vi "FGV System.vi"(0 "Optionen":T2, 1 "Wartungsintervall:":sgl format="%#_5g", 2 "Zeitstempel":timestamp, 3 "Reset BMP":bool, 4 "Reset SQP":bool, 5 "error in (no error)":errorcluster caption="Fehler (Eingang, kein Fehler)", 7 "Werkseinstellung erstellen":T1 caption="Werkseinstellung", 9 "Aktionen":T3) -> (13 "Werkseinstellung erstellen":T1 caption="Werkseinstellung", 14 "Optionen":T2, 15 "Wartungsintervall:":sgl, 16 "Zeitstempel":timestamp, 17 "Reset BMP":bool, 18 "Reset SQP":bool, 19 "error out":errorcluster caption="Fehler (Ausgang)")   [LabVIEW 2020, in "System Einstellungen V2.lvlib"]
uses:
  System Einstellungen V2.lvlib
  Aktioen FGV System.ctl
  Optionen.ctl
  Visualisierungs Elemente/Button.ctl
  SysLog/SysLog Interface.ctl
  Allgemein/allgemeine Sub-VIs.lvlib
  SysLog/SysLog.lvlib
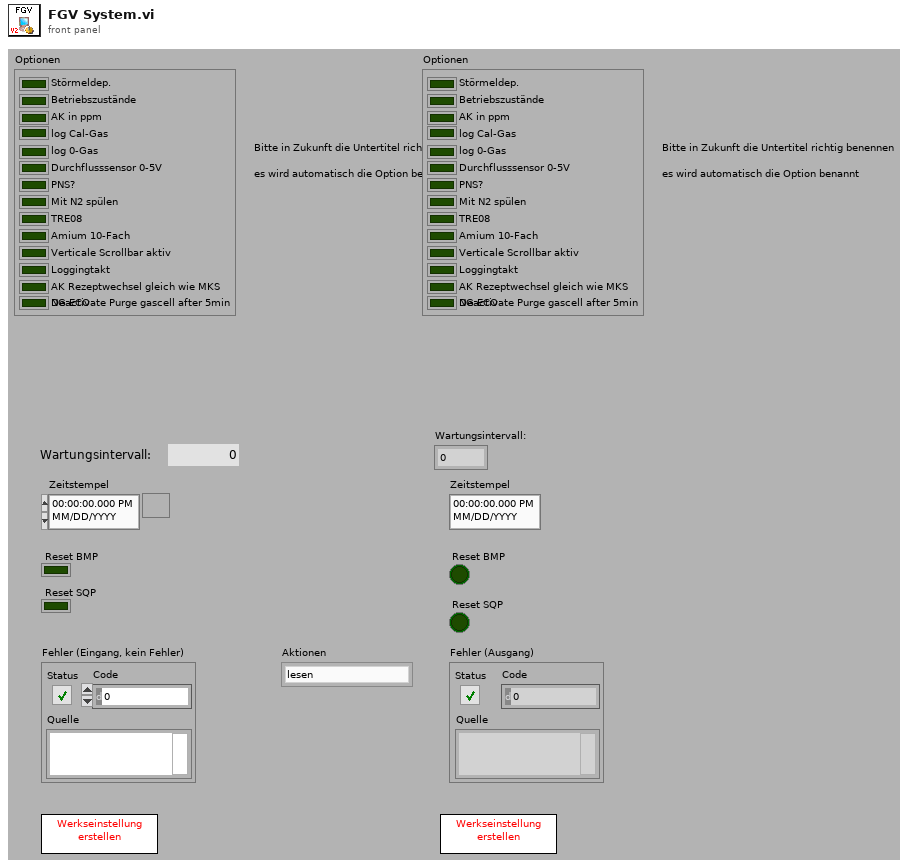
[diagram p1: front panel]
types:
  T1 = typedef "Button.ctl" = bool
  T2 = typedef "System Einstellungen V2.lvlib/Optionen.ctl" = cluster{"Störmeldep.":bool, "Betriebszustände":bool, "AK in ppm":bool, "log Cal-Gas":bool, "log 0-Gas":bool, "Durchflusssensor 0-5V":bool, "PNS?":bool, "Mit N2 spülen":bool, "TRE08":bool, "Amium 10-Fach":bool, "Verticale Scrollbar aktiv":bool, "Loggingtakt":bool, "AK Rezeptwechsel gleich wie MKS":bool, "NG ECO":bool}
  T3 = typedef "System Einstellungen V2.lvlib/Aktioen FGV System.ctl" = enum16{"lesen", "laden", "speichern", "Optionen schreiben", "Zeitstempel", "Reset BMP", "Reset SQP", "Wartung", "Werkseinstellung"}
  T4 = typedef "SysLog.lvlib/SysLog Interface.ctl" = cluster{"FehlermeldungsCode":i32, "ErfolgsmeldungsCode":i32, "ParameterListenString":string, "Anzeige":bool, "SysLogIcon":enum16{"OK", "Warnung", "Fehler"}, "intern":bool}
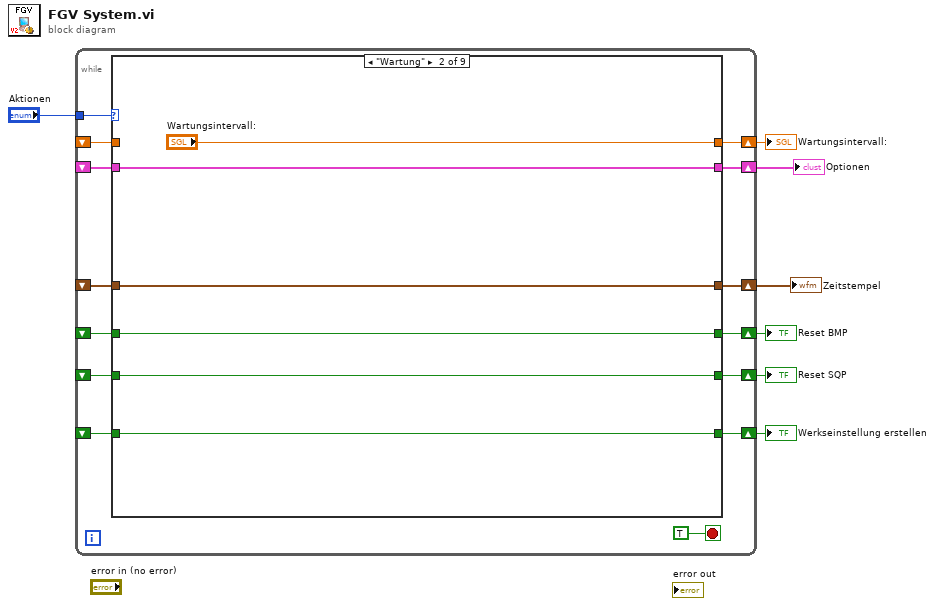
[diagram p0: block diagram]
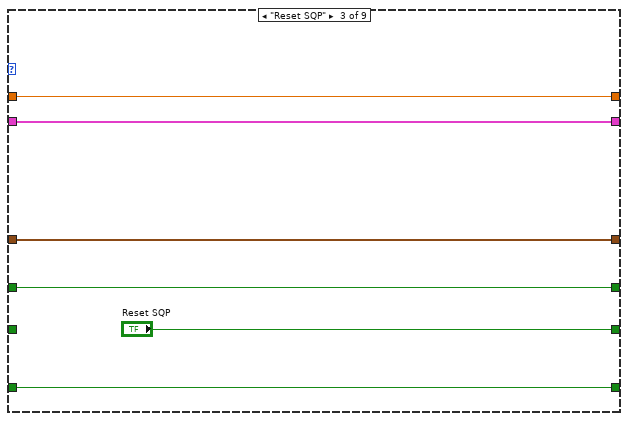
[diagram p3: hidden frame]
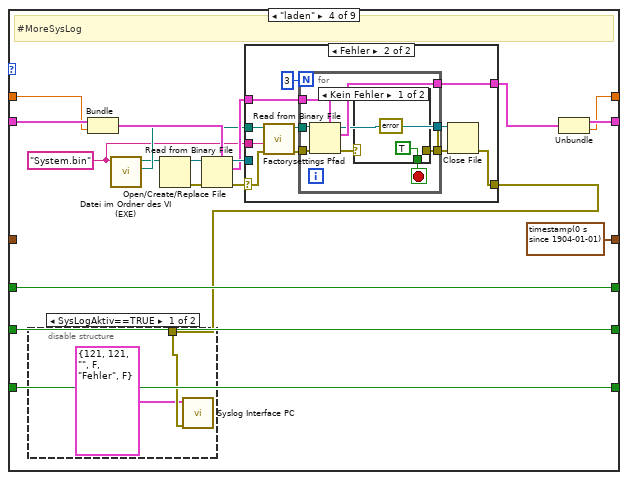
[diagram p4: hidden frame]
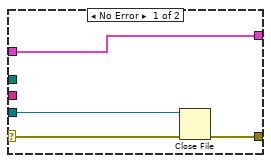
[diagram p5: hidden frame]
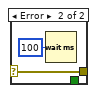
[diagram p6: hidden frame]
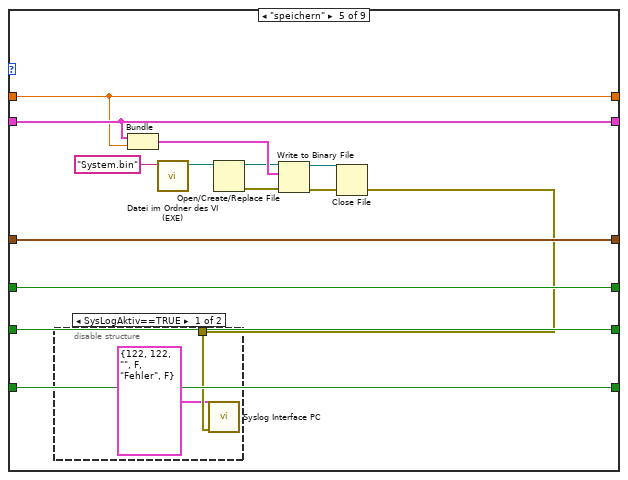
[diagram p8: hidden frame]
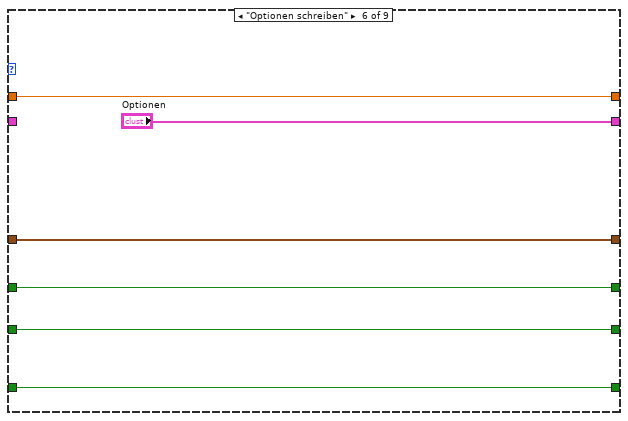
[diagram p10: hidden frame]
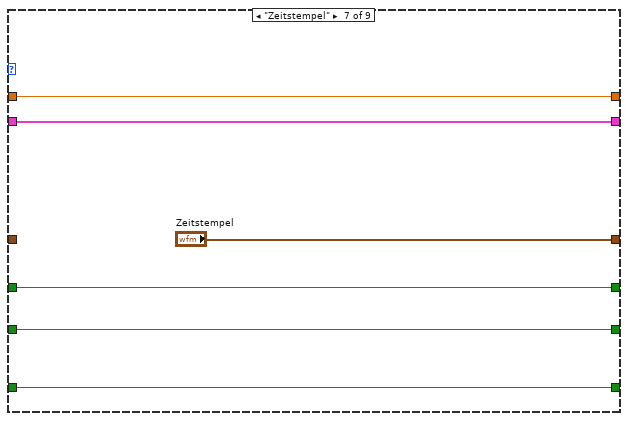
[diagram p11: hidden frame]
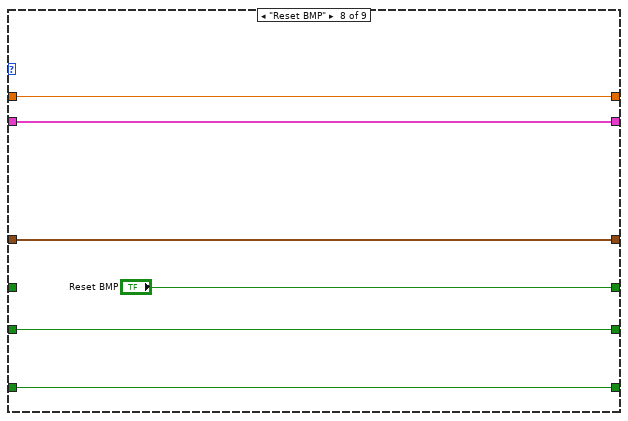
[diagram p12: hidden frame]
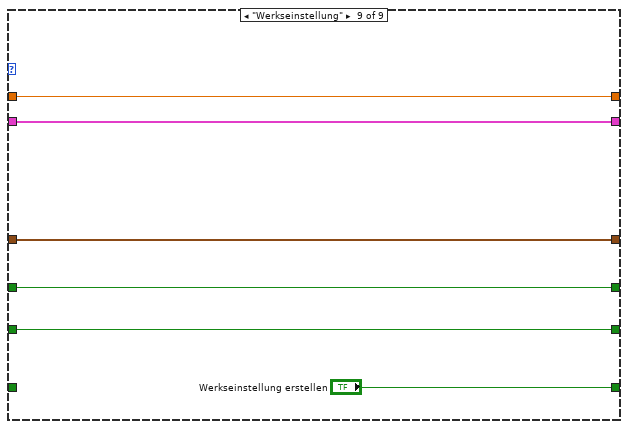
[diagram p13: hidden frame]
diagram:
  n1 = while {
    shift-right: [w18] -> w6
    shift-left: _ -> [w19]
    tunnel: "Aktionen" -> [w20]
    shift-right: [w17] -> w5
    shift-left: _ -> [w16]
    shift-right: [w15] -> w4
    shift-left: _ -> [w14]
    shift-right: [w13] -> w3
    shift-left: _ -> [w12]
    shift-right: [w11] -> w2
    shift-left: _ -> [w10]
    shift-right: [w9] -> w1
    shift-left: _ -> [w8]
    stop <- TRUE stop-if-true
    n2 = case shown="\"Wartung\"" w20 {
      tunnel: w19 -> [w27 w33 w39 w55 w96 _ w114 w121 w126]
      tunnel: [w27 w33 w39 w52 w96 "Optionen" w114 w121 w126] -> w18
      tunnel: [w26 w32 w38 timestamp(0 s since 1904-01-01) ("Zeitstempel") w100 w108 "Zeitstempel" w120 w125] -> w17
      tunnel: w16 -> [w26 w32 w38 _ w100 w108 _ w120 w125]
      tunnel: [w25 w31 w37 w57 w99 w107 w113 "Reset BMP" w124] -> w15
      tunnel: w14 -> [w25 w31 w37 w57 w99 w107 w113 _ w124]
      tunnel: [w24 w30 "Reset SQP" w56 w98 w106 w112 w118 w123] -> w13
      tunnel: w12 -> [w24 w30 _ w56 w98 w106 w112 w118 w123]
      tunnel: [w23 "Wartungsintervall:" w35 w51 w95 w105 w111 w117 w127] -> w11
      tunnel: w10 -> [w23 _ w35 w53 w95 w105 w111 w117 w127]
      tunnel: [w22 w28 w34 w40 w88 w104 w110 w116 "Werkseinstellung erstellen"] -> w9
      tunnel: w8 -> [w22 w28 w34 w40 w88 w104 w110 w116 _]
      frame "lesen", Default {
      }
      frame "Wartung" {
      }
      frame "Reset SQP" {
      }
      frame "laden" {
        w44 = "System.bin" ("Dateiname")
        # "#MoreSysLog"
        n3 = Bundle("Optionen"=w55, "Wartungsintervall:"=w53) -> (w54:cluster{"Optionen":T2, "Wartungsintervall:":sgl})  [unwired: 1 in]
        n4 = call "Datei im Ordner des VI (EXE).vi"("Dateiname"=w44) -> ("Ordner des Haupt-VIs"=w45:path, "Dateipfad im Ordner des Haupt-VIs"=w42:path)  [unwired: 8 in, 1 out]
        n5 = Open/Create/Replace File(file path (use dialog)=w42) -> (refnum out=w41:refnum<file>, error out=w43:errorcluster)  [unwired: 5 in, 1 out]
        n6 = Read from Binary File(5:w54, 8:w43, 11:w41) -> (0:w49:errorcluster, 2:w47:cluster{"Optionen":T2, "Wartungsintervall:":sgl}, 3:w48:refnum<file>)  [unwired: 4 out]
        n7 = case shown="Fehler" w49 {
          selector: w49 -> [w61 w65]
          tunnel: w45 -> [_ w66]
          tunnel: w47 -> [w62 w64]
          tunnel: [w62 w72] -> w46
          tunnel: [w59 w70] -> w50
          tunnel: w48 -> [w60 _]
          tunnel: w44 -> [_ w63]
          frame No Error {
            n8 = Close File(refnum=w60, error in=w61) -> (error out=w59:errorcluster)  [unwired: 1 out]
          }
          frame Error {
            n9 = call "Factorysettings Pfad.vi"("error in (no error)"=w65, "Dateiname"=w63, "Ordner des Haupt-VIs"=w66) -> ("error out"=w67:errorcluster, "Pfad Factorysettings"=w68:path)  [unwired: 7 in]
            n10 = for {
              N: 3 -> [_]
              tunnel: w67 -> [w79]
              tunnel: w68 -> [w78]
              tunnel: [w77] -> w72
              tunnel: [w76] -> w71
              tunnel: [w75] -> w69
              tunnel: w64 -> [w74]
              stop <- w80 stop-if-true
              n11 = Read from Binary File(5:w74, 8:w79, 11:w78) -> (0:w81:errorcluster, 2:w77:cluster{"Optionen":T2, "Wartungsintervall:":sgl}, 3:w75:refnum<file>)  [unwired: 3 in, 1 out]
              n12 = case shown="Kein Fehler" w81 {
                selector: w81 -> [_ w84]
                tunnel: [TRUE _] -> w80
                tunnel: [errorcluster {"status"=FALSE, "code"=0, "source"=""} ("error IO") w84] -> w76
                frame No Error {
                }
                frame Error {
                  n13 = Wait (ms)(milliseconds to wait=u32 100 ("Zu wartende ms")) -> ()  [unwired: 1 out]
                }
              }
            }
            n14 = Close File(refnum=w69, error in=w71) -> (error out=w70:errorcluster)  [unwired: 1 out]
          }
        }
        n15 = disable-structure shown="SysLogAktiv==TRUE" {
          disable-tunnel: w50 -> [w87 _]
          frame condition #0 (active) {
            n16 = call "Syslog Interface PC.vi"("Fehler (in)"=w87, "Cluster (in)"=T4 {"FehlermeldungsCode"=121, "ErfolgsmeldungsCode"=121, "ParameterListenString"="", "Anzeige"=FALSE, "SysLogIcon"=enum."Fehler", "intern"=FALSE}) -> ()  [unwired: 9 in, 1 out]
          }
          frame condition #1 {
          }
        }
        n17 = Unbundle(w46) -> ("Optionen"=w52:T2, "Wartungsintervall:"=w51:sgl)
      }
      frame "speichern" {
        n18 = Bundle("Optionen"=w96, "Wartungsintervall:"=w95) -> (w97:cluster{"Optionen":T2, "Wartungsintervall:":sgl})  [unwired: 1 in]
        n19 = call "Datei im Ordner des VI (EXE).vi"("Dateiname"="System.bin") -> ("Dateipfad im Ordner des Haupt-VIs"=w94:path)  [unwired: 8 in, 2 out]
        n20 = Open/Create/Replace File(file path (use dialog)=w94) -> (refnum out=w93:refnum<file>, error out=w92:errorcluster)  [unwired: 5 in, 1 out]
        n21 = Write to Binary File(file (use dialog)=w93, data=w97, error in=w92) -> (refnum out=w90:refnum<file>, error out=w91:errorcluster)  [unwired: 4 out]
        n22 = Close File(refnum=w90, error in=w91) -> (error out=w89:errorcluster)  [unwired: 1 out]
        n23 = disable-structure shown="SysLogAktiv==TRUE" {
          disable-tunnel: w89 -> [w103 _]
          frame condition #0 (active) {
            n24 = call "Syslog Interface PC.vi"("Fehler (in)"=w103, "Cluster (in)"=T4 {"FehlermeldungsCode"=122, "ErfolgsmeldungsCode"=122, "ParameterListenString"="", "Anzeige"=FALSE, "SysLogIcon"=enum."Fehler", "intern"=FALSE}) -> ()  [unwired: 9 in, 1 out]
          }
          frame condition #1 {
          }
        }
      }
      frame "Optionen schreiben" {
      }
      frame "Zeitstempel" {
      }
      frame "Reset BMP" {
      }
      frame "Werkseinstellung" {
      }
    }
  }
  "Optionen" <- w6
  "Zeitstempel" <- w5
  "Reset BMP" <- w4
  "Reset SQP" <- w3
  "Wartungsintervall:" <- w2
  "Werkseinstellung erstellen" <- w1
